vi "ReadMerecuryIPS_LevelMeter.vi"() -> ()   [LabVIEW 2014]
panel:
  out "Numeric 2":dbl
  out "Numeric":dbl
  in  "error in (no error)":errorcluster
  out "error out":errorcluster
  out "String 4":string
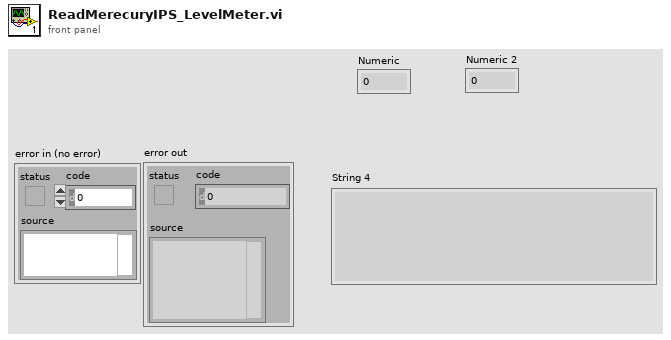
[diagram p1: front panel]
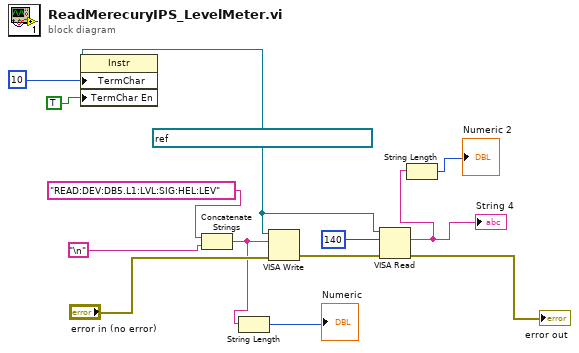
[diagram p0: block diagram]
diagram:
  w4 = refnum<visa-resource-name> "TCPIP0::192.168.128.3::7020::SOCKET" ("VISA resource name")
  n1 = property class="Instr"(reference=w4, "TermChar"=10, "TermChar En"=TRUE) -> ()  [unwired: 1 in, 2 out]
  n2 = Concatenate Strings("READ:DEV:DB5.L1:LVL:SIG:HEL:LEV" ("string"), "\n") -> (w8:string)
  n3 = String Length(string=w8) -> (length=→"Numeric":i32)
  n4 = VISA Write(VISA resource name=w4, write buffer=w8, error in (no error)="error in (no error)") -> (error out=w13:errorcluster)  [unwired: 2 out]
  n5 = VISA Read(VISA resource name=w4, byte count=140, error in (no error)=w13) -> (read buffer=w5:string, error out=→"error out":errorcluster)  [unwired: 2 out]
  "String 4" <- w5
  n6 = String Length(string=w5) -> (length=→"Numeric 2":i32)
